vi "MDAQ_ReadDatfile.vi"(8 "error in":errorcluster, 11 "file path (use dialog)":path) -> (0 "error out":errorcluster, 1 "Run Data Cluster":T1 {"Temperature B" scale=0.0..100.0; "Temperature A" scale=0.0..100.0}, 2 "Run Info Out":T2)   [LabVIEW 2021]
uses:
  XML_Cluster.ctl
  DAT_Cluster.ctl
  <vilib>/Utility/error.llb/DialogType.ctl
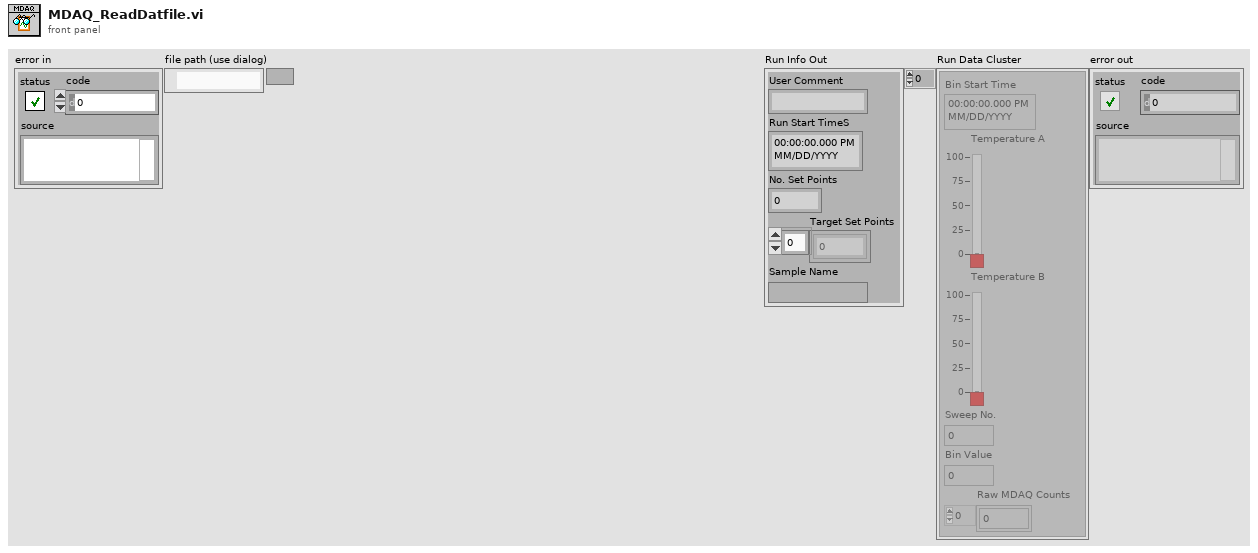
[diagram p1: front panel]
types:
  T1 = typedef "DAT_Cluster.ctl" = cluster{"Bin Start Time":timestamp, "Temperature A":dbl, "Temperature B":dbl, "Sweep No.":i32, "Bin Value":i32, "Raw MDAQ Counts":i32[]}[]
  T2 = typedef "XML_Cluster.ctl" = cluster{"User Comment":string, "Run Start TimeS":timestamp, "No. Set Points":u32, "Target Set Points":i32[], "Sample Name":string}
  T3 = typedef "DialogType.ctl" = u16
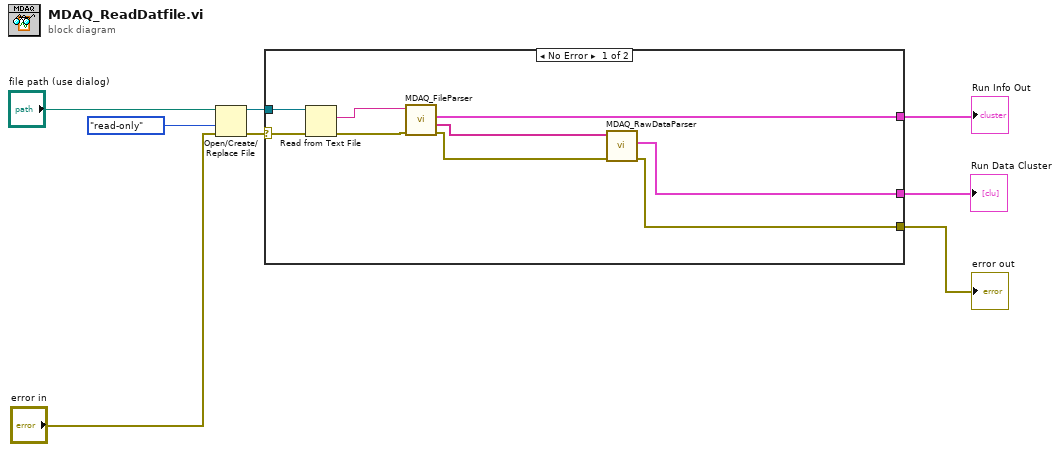
[diagram p0: block diagram]
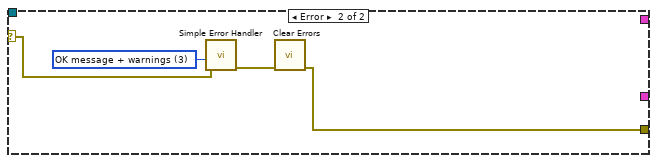
[diagram p2: hidden frame]
diagram:
  n1 = Open/Create/Replace File(file path (use dialog)="file path (use dialog)", error in="error in", access (0:read/write)=enum16{"read/write", "read-only", "write-only"}."read-only") -> (refnum out=w4:refnum<file>, error out=w5:errorcluster)  [unwired: 3 in, 1 out]
  n2 = case shown="No Error" w5 {
    selector: w5 -> [w16 w20]
    tunnel: w4 -> [w17 _]
    tunnel: [w11 _] -> w3
    tunnel: [w10 _] -> w2
    tunnel: [w9 w18] -> w1
    frame No Error {
      n3 = Read from Text File(file (use dialog)=w17, error in=w16) -> (text=w15:string, error out=w14:errorcluster)  [unwired: 2 in, 2 out]
      n4 = call "MDAQ_FileParser.vi"("error in"=w14, "ReadData"=w15) -> ("error out"=w12:errorcluster, "Raw Data"=w13:string[], "Run Info"=w11:T2)  [unwired: 7 in]
      n5 = call "MDAQ_RawDataParser.vi"("error in"=w12, "Raw Data In"=w13) -> ("error out"=w9:errorcluster, "Run Data Cluster"=w10:T1)  [unwired: 8 in]
    }
    frame Error {
      w21 = T3 3 items=["no dialog", "OK message", "continue or stop message", "OK message + warnings", "continue/stop + warnings"] ("type of dialog (OK msg:1)")
      n6 = call <vilib>:"Simple Error Handler.vi"("type of dialog (OK msg:1)"=w21, "error in (no error)"=w20) -> ("error out"=w19:errorcluster)  [unwired: 3 in, 4 out]
      n7 = call <vilib>:"Clear Errors.vi"("error in (no error)"=w19) -> ("error out"=w18:errorcluster)  [unwired: 5 in, 1 out]
    }
  }
  "Run Data Cluster" <- w2
  "Run Info Out" <- w3
  "error out" <- w1
